vi "PDP.vi"() -> ()   [LabVIEW 2019]
doc: "This VI represents about 90% of the user interface, the remainder consisting of the various pop-up windows.\nA diagram of the NMR system is presented, with buttons to represent each component. Parameters may be changed by pressing one of these buttons, which results in messages being passed to one of several other, high-level VIs whose job it is to take action. After such action is taken, messages may be passed back to this VI, indicating new data to be displayed on the front panel."
uses:
  PDP Global.vi
  TPS Global.vi
  <vilib>/Utility/config.llb/Read Key (Path).vi
  <vilib>/Utility/config.llb/NI_LVConfig.lvlib
panel:
  in  "sel_auto_sw":bool[](array[boolean])=[TRUE, TRUE, TRUE, FALSE, FALSE, FALSE]
  in  "auto_switch_NMR_chan":bool caption="NMR channel \nauto switching"
  in  "RF Off":bool
  in  "RF On":bool
  in  "Mon. Time":i32=30
  out "Polysub Signal":cluster{"x-Axis":dbl[], "Signal":dbl[]}(graph)
  out "CarbGlass":dbl=9.54
  out "Bottom Chip":dbl=9.54
  out "Top Chip":dbl=9.54
  out "NMR Tune Light":bool
  in  "NMR Tune":bool
  out "Clear Message Time":i32
  in  "DC Convert":bool
  out "Bot Plat (K)":dbl=nan format="%.1f"
  out "Top Plat (K)":dbl=nan format="%.1f"
  in  "Submit Comment":bool
  in  "User Comment (press submit when done)":string
  in  "Stop NMR Sweep":bool
  in  "Enable TCL Buttons":bool
  in  "NewEventFile":bool
  in  "NewBaseFile":bool
  out "Separator Flow":dbl=10.0 format="%.1f"
  out "Main Flow":dbl=9.83 format="%.1f"
  in  "Beep on Update":bool
  out "Raw & Base":cluster{"x-Axis":dbl[], "Signal":dbl[]}[](graph)
  in  "5 min":bool
  out "History Plot":cluster{dbl, dbl}[](graph)
  out "Event Number":i32=-15
  in  "Scan Freq":i32=100
  in  "ScanSteps":i32=500
  in  "RF Power":i32=280
  in  "RF Mod":i32=400
  in  "Sweeps":i32=100
  in  "RF Freq":dbl=213.0 format="%.3f"
  in  "Yale Gain":i32(listbox)
  in  "Decrease":bool
  in  "Increase":bool
  in  "Up":bool
  in  "Down":bool
  in  "+1 hour":bool
  in  "30 min":bool
  in  "15 min":bool
  out "Polarization (%)":string="-13.06%"
  out "Monitor Light":bool
  in  "Monitor":bool
  out "Take Data Light":bool
  out "Pause Light":bool=TRUE
  out "QMeter":string="Bot Proton NH3"
  in  "Error":bool
  out "3He Pressure":dbl=9.83 format="%.3f"
  out "4He Pressure":dbl=-0.06 format="%.3f"
  out "Timestamp":string="06May1999  19h28m14s"
  in  "Init QCA":bool
  out "PolyFit Area (arb units)":dbl=-14.751 format="%.8f"
  out "User Message":string="Message: 23Jul2001  15h39m59s\nQCA Module Started"
  in  "Cal. Const.":dbl=0.64413 format="%.6f"
  out "Update At (sec)":dbl=2147483647.0
  out "Next Update":dbl=1151566443.0 format="%.1f"
  in  "Baseline":bool
  out "Subtracted Signal & PolyFit Curve":cluster{"x-Axis":dbl[], "Signal":dbl[]}[](graph)
  out "3He Temp":dbl=1.023 format="%.2f"
  out "4He Temp":dbl=nan format="%.2f"
  in  "Save Channel List":bool
  in  "NMR Channel":i32(listbox)
  in  "Previous Messages":u16(ring)
  in  "Take Data":bool
  in  "One Point":bool
  in  "Pause":bool
  # "PDP:  Polarization Display Panel"
  # "Data for Last Event Displayed:"
  # "RF Output"
  # "X-Axis"
  # "Temp (K)"
  # "Press (Torr)"
  # "4He"
  # "Y-Axis"
  # "3He"
  # "Top"
  # "Bottom"
  # "Chip (W)"
  # "Plat (K)"
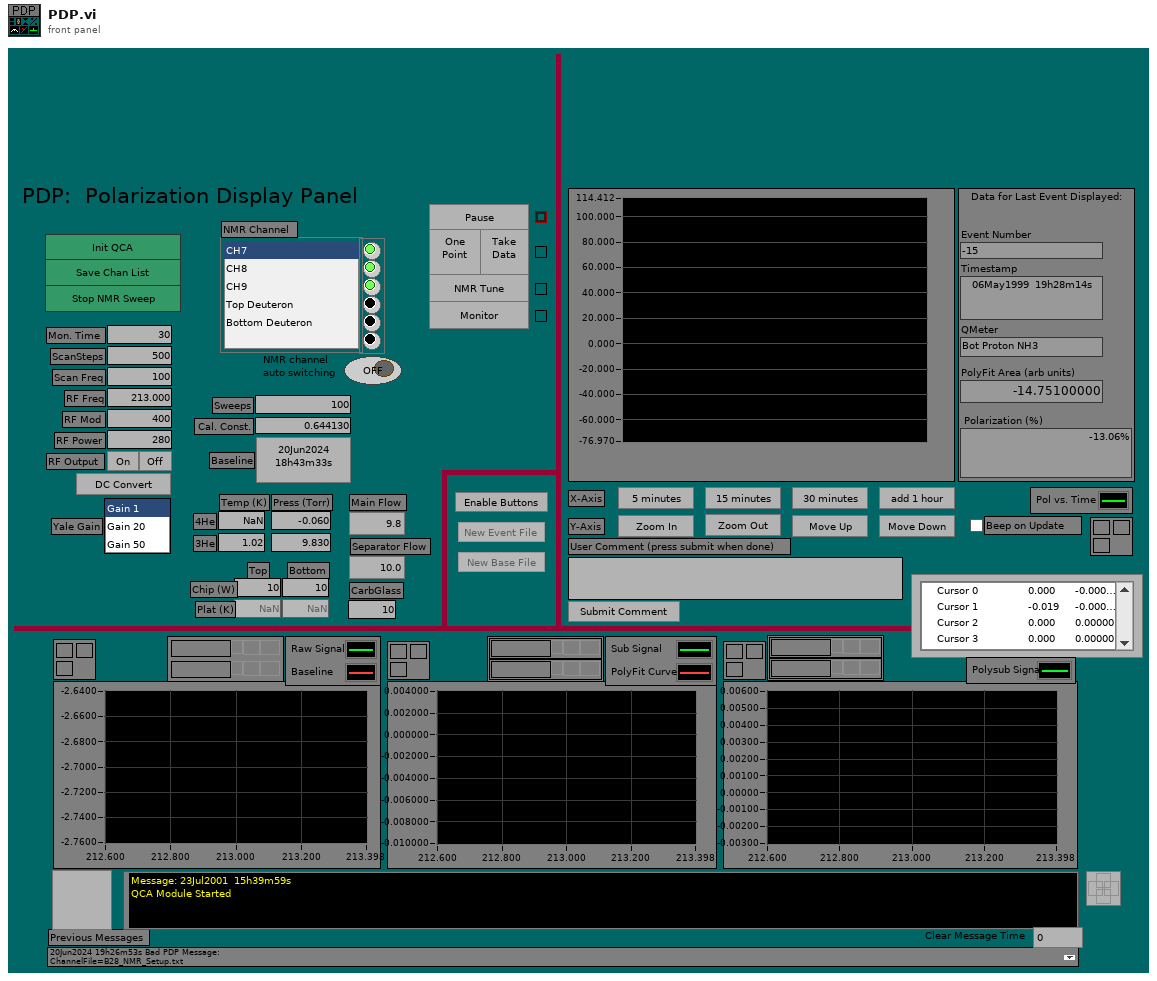
[diagram p1: front panel]
types:
  T1 = enum16{"No Message", "Bad Message", "RFFreq=", "RFMod=", "RFPower=", "QMeterName=", "YaleGain=", "ScanSweeps=", "ScanSteps=", "ScanFreq=", "Material=", "Baseline=", "CalConst=", "MonitorDelay=", "Channel=", "Channels=", "QCAPause", "QCATakeData", "QCANMRTune", "QCAMonitor", "Timer=", "LeadCurrent=", "LeadVoltage=", "MagCurrent=", "MagField=", "MagStatus=", "Setpoint=", "Setrate=", "HeaterDelay=", "Heater=", "HeaterDialog", "MagRemote", "MagLocal", "SendHe4Range", "uWaveFreq=", "uWavePower=", "BellowsPos=", "Event=", "Beep", "Message=", "Warning=", "Error=", "Address=", "Stop"}
  T2 = typedef "NI_LVConfig.lvlib/Config Data RefNum.ctl" = refnum<k1>
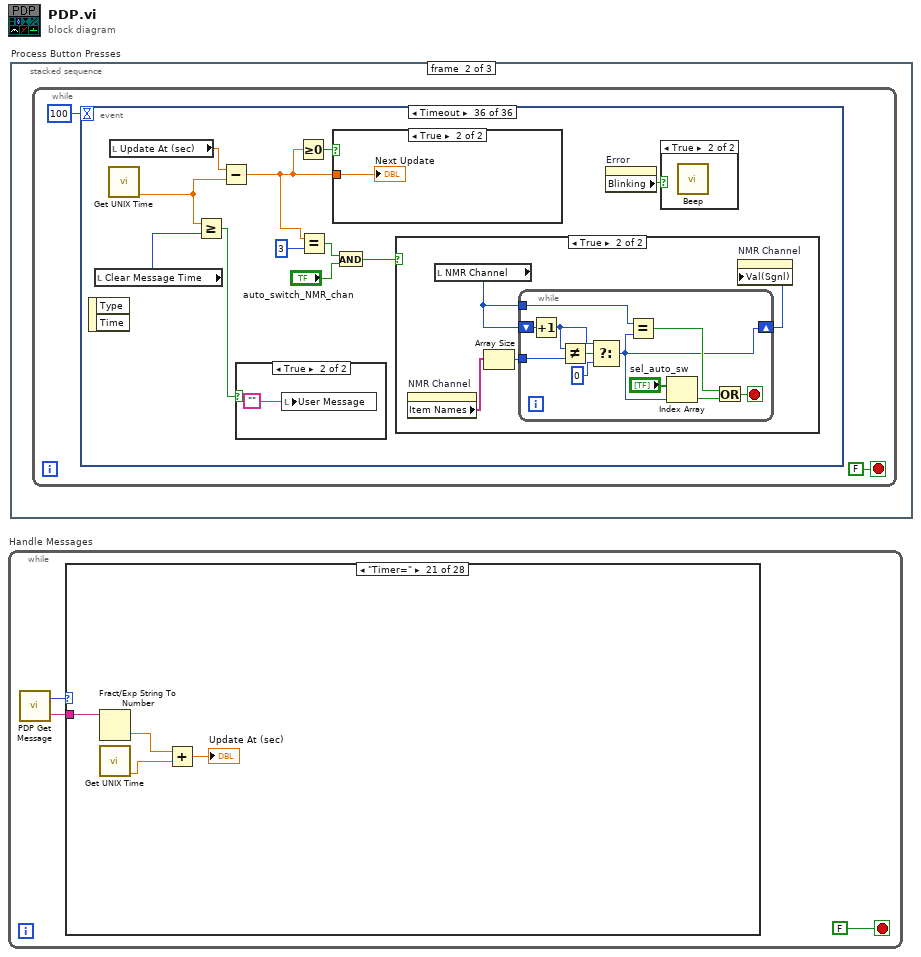
[diagram p0: block diagram]
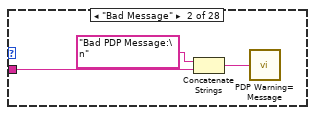
[diagram p3: hidden frame]
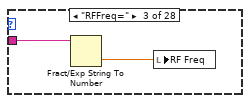
[diagram p4: hidden frame]
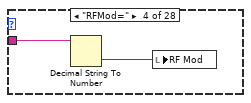
[diagram p5: hidden frame]
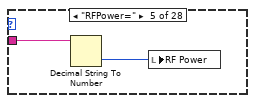
[diagram p6: hidden frame]
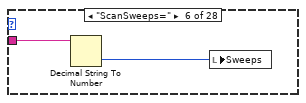
[diagram p7: hidden frame]
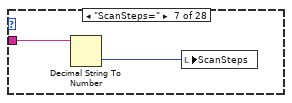
[diagram p8: hidden frame]
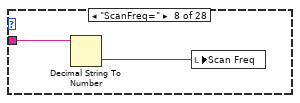
[diagram p9: hidden frame]
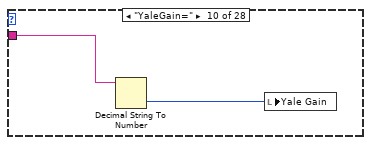
[diagram p11: hidden frame]
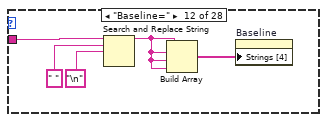
[diagram p13: hidden frame]
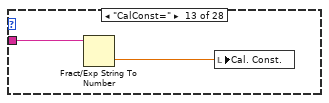
[diagram p14: hidden frame]
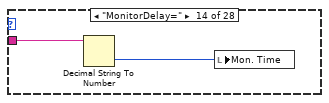
[diagram p15: hidden frame]
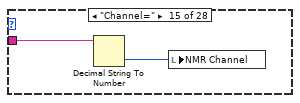
[diagram p16: hidden frame]
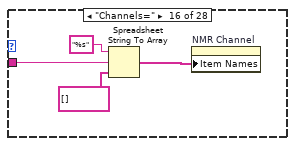
[diagram p17: hidden frame]
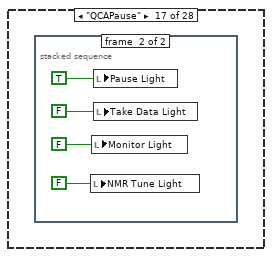
[diagram p18: hidden frame]
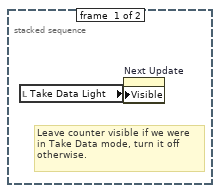
[diagram p19: hidden frame]
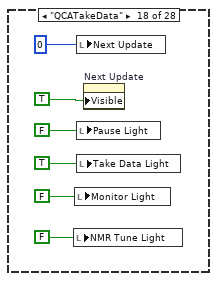
[diagram p20: hidden frame]
diagram:
  n1 = while "Handle Messages" {
    stop <- FALSE stop-if-true
    n2 = call "PDP Get Message.vi"() -> ("PDP Message Type"=w2:T1, "Text"=w3:string)  [unwired: 1 in]
    n3 = case shown="\"Timer=\"" w2 {
      tunnel: w3 -> [_ w4 w8 w10 w12 w14 w16 w18 _ w20 _ w24 w27 w29 w31 w32 _ _ _ _ w61 w62 _ w256 w270 w285 w298 _]
      frame "No Message", Default {
      }
      frame "Bad Message" {
        n4 = Concatenate Strings("Bad PDP Message:\n" ("Message"), w4) -> (w5:string)
        n5 = call "PDP Warning= Message.vi"("Message"=w5) -> ()
      }
      frame "RFFreq=" {
        n6 = Fract/Exp String To Number(string=w8) -> (number=w7:dbl)  [unwired: 3 in, 1 out]
        n7 = local write "RF Freq"(w7) -> ()
      }
      frame "RFMod=" {
        n8 = Decimal String To Number(string=w10) -> (number=w9:i32)  [unwired: 2 in, 1 out]
        n9 = local write "RF Mod"(w9) -> ()
      }
      frame "RFPower=" {
        n10 = Decimal String To Number(string=w12) -> (number=w11:i32)  [unwired: 2 in, 1 out]
        n11 = local write "RF Power"(w11) -> ()
      }
      frame "ScanSweeps=" {
        n12 = Decimal String To Number(string=w14) -> (number=w13:i32)  [unwired: 2 in, 1 out]
        n13 = local write "Sweeps"(w13) -> ()
      }
      frame "ScanSteps=" {
        n14 = Decimal String To Number(string=w16) -> (number=w15:i32)  [unwired: 2 in, 1 out]
        n15 = local write "ScanSteps"(w15) -> ()
      }
      frame "ScanFreq=" {
        n16 = Decimal String To Number(string=w18) -> (number=w17:i32)  [unwired: 2 in, 1 out]
        n17 = local write "Scan Freq"(w17) -> ()
      }
      frame "QMeterName=" {
      }
      frame "YaleGain=" {
        n18 = Decimal String To Number(string=w20) -> (number=w19:i32)  [unwired: 2 in, 1 out]
        n19 = local write "Yale Gain"(w19) -> ()
      }
      frame "Material=" {
      }
      frame "Baseline=" {
        n20 = Search and Replace String(input string=w24, search string=" ", replace string="\n" ("replace string (\"\")")) -> (result string=w21:string)  [unwired: 5 in, 3 out]
        n21 = Build Array(w21, w21, w21, w21) -> (w25:string[])
        n22 = property on="Baseline" class="Bool"("Strings [4]"=w25) -> ()  [unwired: 2 in, 2 out]
      }
      frame "CalConst=" {
        n23 = Fract/Exp String To Number(string=w27) -> (number=w26:dbl)  [unwired: 3 in, 1 out]
        n24 = local write "Cal. Const."(w26) -> ()
      }
      frame "MonitorDelay=" {
        n25 = Decimal String To Number(string=w29) -> (number=w28:i32)  [unwired: 2 in, 1 out]
        n26 = local write "Mon. Time"(w28) -> ()
      }
      frame "Channel=" {
        n27 = Decimal String To Number(string=w31) -> (number=w30:i32)  [unwired: 2 in, 1 out]
        n28 = local write "NMR Channel"(w30) -> ()
      }
      frame "Channels=" {
        n29 = Spreadsheet String To Array(format string="%s", spreadsheet string=w32, array type (2D Dbl)=string[] []) -> (array=w34:string[])  [unwired: 1 in]
        n30 = property on="NMR Channel" class="LstBox (strict)"("Item Names"=w34) -> ()  [unwired: 2 in, 2 out]
      }
      frame "QCAPause" {
        n31 = stacked-sequence {
          frame #0 {
            # "Leave counter visible if we were\nin Take Data mode, turn it off\notherwise."
            n32 = local read "Take Data Light"() -> (w36:bool)
            n33 = property on="Next Update" class="DigNum (strict)"("Visible"=w36) -> ()  [unwired: 2 in, 2 out]
          }
          frame #1 {
            n34 = local write "NMR Tune Light"(FALSE ("NMR Tune Light")) -> ()
            n35 = local write "Monitor Light"(FALSE ("Cont Sweep Light")) -> ()
            n36 = local write "Pause Light"(TRUE ("Pause Light")) -> ()
            n37 = local write "Take Data Light"(FALSE ("Take Data Light")) -> ()
          }
        }
      }
      frame "QCATakeData" {
        n38 = local write "NMR Tune Light"(FALSE ("NMR Tune Light")) -> ()
        n39 = local write "Monitor Light"(FALSE ("Cont Sweep Light")) -> ()
        n40 = local write "Next Update"(0 ("Next Update")) -> ()
        n41 = local write "Pause Light"(FALSE ("Pause Light")) -> ()
        n42 = local write "Take Data Light"(TRUE ("Take Data Light")) -> ()
        n43 = property on="Next Update" class="DigNum (strict)"("Visible"=TRUE) -> ()  [unwired: 2 in, 2 out]
      }
      frame "QCANMRTune" {
        n44 = local write "NMR Tune Light"(TRUE ("NMR Tune Light")) -> ()
        n45 = local write "Monitor Light"(FALSE ("Cont Sweep Light")) -> ()
        n46 = local write "Pause Light"(FALSE ("Pause Light")) -> ()
        n47 = local write "Take Data Light"(FALSE ("Take Data Light")) -> ()
        n48 = property on="Next Update" class="DigNum (strict)"("Visible"=FALSE) -> ()  [unwired: 2 in, 2 out]
      }
      frame "QCAMonitor" {
        n49 = local write "NMR Tune Light"(FALSE ("NMR Tune Light")) -> ()
        n50 = local write "Monitor Light"(TRUE ("Cont Sweep Light")) -> ()
        n51 = local write "Next Update"(0 ("Next Update")) -> ()
        n52 = local write "Pause Light"(FALSE ("Pause Light")) -> ()
        n53 = local write "Take Data Light"(FALSE ("Take Data Light")) -> ()
        n54 = property on="Next Update" class="DigNum (strict)"("Visible"=TRUE) -> ()  [unwired: 2 in, 2 out]
      }
      frame "Timer=" {
        n55 = Fract/Exp String To Number(string=w61) -> (number=w60:dbl)  [unwired: 3 in, 1 out]
        n56 = call "Get UNIX Time.vi"() -> ("UNIX_seconds_dbl"=w58:dbl)  [unwired: 10 in, 1 out]
        n57 = Add(x=w60, y=w58) -> (x+y=→"Update At (sec)":dbl)
      }
      frame "Event=" {
        n58 = Unflatten From String(type=string[][] [], binary string=w62) -> (value=w64:string[][])  [unwired: 3 in, 2 out]
        n59 = stacked-sequence {
          tunnel: w64 -> [w75 w103 w124 w131 w134 w138 w165 w168 w173 w177 w181 w186 w197 w206 w209 w215 w224 w233 w237 w243 _ w251]
          frame #0 {
            # "Set the X axis of the signal plots."
            n60 = call "Text Get Event Fragment.vi"("Event"=w75, "Fragment Type"="RFFreq") -> ("Fragment"=w80:string)  [unwired: 1 out]
            n61 = call "Text Get Event Fragment.vi"("Event"=w75, "Fragment Type"="RFMod") -> ("Fragment"=w81:string)  [unwired: 1 out]
            n62 = call "Text Get Event Fragment.vi"("Event"=w75, "Fragment Type"="ScanSteps") -> ("Fragment"=w77:string)  [unwired: 1 out]
            n63 = global read "PDP Global.vi" "Last Mod"() -> (w71:dbl)
            n64 = global read "PDP Global.vi" "Last Freq"() -> (w74:dbl)
            n65 = global read "PDP Global.vi" "Last Steps"() -> (w72:i32)
            n66 = Fract/Exp String To Number(string=w80) -> (number=w73:dbl)  [unwired: 3 in, 1 out]
            n67 = Decimal String To Number(string=w81) -> (number=w79:i32)  [unwired: 2 in, 1 out]
            n68 = Decimal String To Number(string=w77) -> (number=w69:i32)  [unwired: 2 in, 1 out]
            n69 = Divide(x=w79, y=1000) -> (x/y=w70:dbl)
            n70 = Not Equal?(x=w74, y=w73) -> (x != y?=w66:bool)
            n71 = Not Equal?(x=w71, y=w70) -> (x != y?=w67:bool)
            n72 = Not Equal?(x=w72, y=w69) -> (x != y?=w68:bool)
            n73 = Compound Arithmetic op=OR(w66, w67, w68) -> (w65:bool)
            n74 = case shown="True" w65 {
              tunnel: w69 -> [_ w86]
              tunnel: w70 -> [_ w85]
              tunnel: w73 -> [_ w84]
              frame False {
              }
              frame True {
                n75 = global write "PDP Global.vi" "Last Mod"(w85) -> ()
                n76 = global write "PDP Global.vi" "Last Freq"(w84) -> ()
                n77 = global write "PDP Global.vi" "Last Steps"(w86) -> ()
                n78 = for {
                  N: w86 -> [_]
                  tunnel: [w94] -> w89 mode=indexing
                  i -> [w94]
                }
                n79 = Multiply(x=w89, y=2) -> (x*y=w90:i32[])
                n80 = Divide(x=w90, y=w86) -> (x/y=w93:dbl[])
                n81 = Decrement(x=w93) -> (x-1=w87:dbl[])
                n82 = Multiply(x=w85, y=w87) -> (x*y=w92:dbl[])
                n83 = Add(x=w84, y=w92) -> (x+y=w91:dbl[])
                n84 = global write "PDP Global.vi" "x-Axis"(w91) -> ()
              }
            }
          }
          frame #1 {
            # "Display the Raw Signal and the Baseline Signal."
            n85 = call "Text Get Event Fragment.vi"("Event"=w103, "Fragment Type"="RawSignal") -> ("Fragment"=w102:string)  [unwired: 1 out]
            n86 = call "Text Get Event Fragment.vi"("Event"=w103, "Fragment Type"="BaseSignal") -> ("Fragment"=w101:string)  [unwired: 1 out]
            n87 = global read "PDP Global.vi" "x-Axis"() -> (w99:dbl[])
            n88 = call "String 2 Signal.vi"("String"=w102) -> ("Signal"=w96:dbl[])
            n89 = call "String 2 Signal.vi"("String"=w101) -> ("Signal"=w98:dbl[])
            n90 = Array Size(array=w98) -> (size(s)=w100:i32)
            n91 = Greater Than 0?(x=w100) -> (x > 0?=w95:bool)
            n92 = case shown="True" w95 {
              tunnel: w99 -> [w109 w110]
              tunnel: w98 -> [_ w115]
              tunnel: [w106 w112] -> w97
              tunnel: w96 -> [w108 w111]
              frame False {
                n93 = Bundle("x-Axis"=w109, "Signal"=w108) -> (w107:cluster{"x-Axis":dbl[], "Signal":dbl[]})  [unwired: 1 in]
                n94 = Build Array(w107) -> (w106:cluster{"x-Axis":dbl[], "Signal":dbl[]}[])
              }
              frame True {
                n95 = Bundle("x-Axis"=w110, "Signal"=w111) -> (w114:cluster{"x-Axis":dbl[], "Signal":dbl[]})  [unwired: 1 in]
                n96 = Bundle("x-Axis"=w110, "Signal"=w115) -> (w113:cluster{"x-Axis":dbl[], "Signal":dbl[]})  [unwired: 1 in]
                n97 = Build Array(w114, w113) -> (w112:cluster{"x-Axis":dbl[], "Signal":dbl[]}[])
              }
            }
            "Raw & Base" <- w97
          }
          frame #2 {
            # "Display the Subtracted Signal and the Polyfit Curve."
            n98 = call "Text Get Event Fragment.vi"("Event"=w124, "Fragment Type"="SubSignal") -> ("Fragment"=w122:string)  [unwired: 1 out]
            n99 = call "Text Get Event Fragment.vi"("Event"=w124, "Fragment Type"="PolyCurve") -> ("Fragment"=w123:string)  [unwired: 1 out]
            n100 = global read "PDP Global.vi" "x-Axis"() -> (w119:dbl[])
            n101 = call "String 2 Signal.vi"("String"=w122) -> ("Signal"=w116:dbl[])
            n102 = call "String 2 Signal.vi"("String"=w123) -> ("Signal"=w120:dbl[])
            n103 = Bundle("x-Axis"=w119, "Signal"=w116) -> (w117:cluster{"x-Axis":dbl[], "Signal":dbl[]})  [unwired: 1 in]
            n104 = Bundle("x-Axis"=w119, "Signal"=w120) -> (w118:cluster{"x-Axis":dbl[], "Signal":dbl[]})  [unwired: 1 in]
            n105 = Build Array(w117, w118) -> (→"Subtracted Signal & PolyFit Curve":cluster{"x-Axis":dbl[], "Signal":dbl[]}[])
          }
          frame #3 {
            # "Display the Polysubtracted Signal."
            n106 = call "Text Get Event Fragment.vi"("Event"=w131, "Fragment Type"="PolySignal") -> ("Fragment"=w128:string)  [unwired: 1 out]
            n107 = global read "PDP Global.vi" "x-Axis"() -> (w130:dbl[])
            n108 = call "String 2 Signal.vi"("String"=w128) -> ("Signal"=w127:dbl[])
            n109 = Bundle("x-Axis"=w130, "Signal"=w127) -> (→"Polysub Signal":cluster{"x-Axis":dbl[], "Signal":dbl[]})  [unwired: 1 in]
          }
          frame #4 {
            # "Display the Polysubtracted Signal."
            n110 = call "Text Get Event Fragment.vi"("Event"=w134, "Fragment Type"="Area") -> ("Fragment"=w135:string)  [unwired: 1 out]
            n111 = Fract/Exp String To Number(string=w135) -> (number=→"PolyFit Area (arb units)":dbl)  [unwired: 3 in, 1 out]
          }
          frame #5 {
            # "Display the Polysubtracted Signal."
            n112 = call "Text Get Event Fragment.vi"("Event"=w138, "Fragment Type"="Polarization") -> ("Fragment"=w144:string, "Found"=w137:bool)
            n113 = call "Text Get Event Fragment.vi"("Event"=w138, "Fragment Type"="EventNum") -> ("Fragment"=w140:string)  [unwired: 1 out]
            n114 = Decimal String To Number(string=w140) -> (number=w139:i32)  [unwired: 2 in, 1 out]
            n115 = Fract/Exp String To Number(string=w144) -> (number=w142:dbl)  [unwired: 3 in, 1 out]
            n116 = case shown="True" w137 {
              tunnel: w142 -> [_ w146]
              tunnel: w139 -> [_ w150]
              frame False {
                n117 = local write "Polarization (%)"("") -> ()
              }
              frame True {
                n118 = call "UNIX to LabVIEW.vi"("UNIX Time"=w150) -> ("LabVIEW Time"=w151:dbl)
                n119 = Absolute Value(x=w146) -> (abs(x)=w149:dbl)
                n120 = property on="History Plot" class="XYGraph (strict)"() -> ("X Scale.Range:Maximum"=w154:dbl, "X Scale.Range:Minimum"=w157:dbl)  [unwired: 2 in, 2 out]
                n121 = Less?(x=w149, y=101.0) -> (x < y?=w147:bool)
                n122 = Format Into String(format string="%+6.1f%", w146) -> (resulting string=→"Polarization (%)":string)  [unwired: 2 in, 1 out]
                n123 = case shown="True" w147 {
                  tunnel: w151 -> [_ w160]
                  tunnel: w146 -> [_ w159]
                  frame False {
                    # "Glitch Signal - don't plot in strip chart"
                  }
                  frame True {
                    n124 = local read "History Plot"() -> (w163:cluster{dbl, dbl}[])
                    n125 = Bundle("LabVIEW Time"=w160, w159) -> (w161:cluster{"LabVIEW Time":dbl, dbl})  [unwired: 1 in]
                    n126 = Build Array (concatenate)(w161, w163) -> (→"History Plot":cluster{"LabVIEW Time":dbl, dbl}[])
                  }
                }
                n127 = Subtract(x=w151, y=w154) -> (x-y=w158:dbl)
                n128 = Compound Arithmetic op=ADD(w158, w154) -> (w156:dbl)
                n129 = Compound Arithmetic op=ADD(w158, w157) -> (w155:dbl)
                n130 = property on="History Plot" class="XYGraph (strict)"("X Scale.Range:Maximum"=w156, "X Scale.Range:Minimum"=w155) -> ()  [unwired: 2 in, 2 out]
              }
            }
          }
          frame #6 {
            # "Display the Polysubtracted Signal."
            n131 = call "Text Get Event Fragment.vi"("Event"=w165, "Fragment Type"="QMeterName") -> ("Fragment"=→"QMeter":string)  [unwired: 1 out]
          }
          frame #7 {
            n132 = call "Text Get Event Fragment.vi"("Event"=w168, "Fragment Type"="EventNum") -> ("Fragment"=w169:string)  [unwired: 1 out]
            n133 = Decimal String To Number(string=w169) -> (number=w167:i32)  [unwired: 2 in, 1 out]
            "Event Number" <- w167
            n134 = call "UNIX to Timestamp.vi"("Seconds"=w167) -> ("Timestamp String"=→"Timestamp":string)
          }
          frame #8 {
            # "Display the Polysubtracted Signal."
            n135 = call "Text Get Event Fragment.vi"("Event"=w173, "Fragment Type"="He3Press") -> ("Fragment"=w174:string)  [unwired: 1 out]
            n136 = Fract/Exp String To Number(string=w174) -> (number=→"3He Pressure":dbl)  [unwired: 3 in, 1 out]
          }
          frame #9 {
            # "Display the Polysubtracted Signal."
            n137 = call "Text Get Event Fragment.vi"("Event"=w177, "Fragment Type"="He3Temp") -> ("Fragment"=w178:string)  [unwired: 1 out]
            n138 = Fract/Exp String To Number(string=w178) -> (number=→"3He Temp":dbl)  [unwired: 3 in, 1 out]
          }
          frame #10 {
            # "Display the Polysubtracted Signal."
            n139 = call "Text Get Event Fragment.vi"("Event"=w181, "Fragment Type"="He4Press") -> ("Fragment"=w182:string)  [unwired: 1 out]
            n140 = Fract/Exp String To Number(string=w182) -> (number=→"4He Pressure":dbl)  [unwired: 3 in, 1 out]
          }
          frame #11 {
            # "Display the Polysubtracted Signal."
            n141 = call "Text Get Event Fragment.vi"("Event"=w186, "Fragment Type"="He4Temp") -> ("Fragment"=w187:string, "Found"=w184:bool)
            n142 = Fract/Exp String To Number(string=w187) -> (number=w185:dbl)  [unwired: 3 in, 1 out]
            n143 = case shown="True" w184 {
              tunnel: w185 -> [_ w189]
              frame False {
              }
              frame True {
                "4He Temp" <- w189
              }
            }
          }
          frame #12 {
            # "Display the Polysubtracted Signal."
            n144 = call "Text Get Event Fragment.vi"("Event"=w197, "Fragment Type"="TopPlat") -> ("Fragment"=w192:string)  [unwired: 1 out]
            n145 = Fract/Exp String To Number(string=w192) -> (number=w191:dbl)  [unwired: 3 in, 1 out]
            "Top Plat (K)" <- w191
            n146 = Less?(x=w191, y=49.0) -> (x < y?=w196:bool)
            n147 = Select(t=2, s=w196, f=0) -> (s? t:f=w193:i32)
            n148 = property on="Top Plat (K)" class="DigNum (strict)"("Disabled"=w193) -> ()  [unwired: 2 in, 2 out]
          }
          frame #13 {
            # "Display the Polysubtracted Signal."
            n149 = call "Text Get Event Fragment.vi"("Event"=w206, "Fragment Type"="BotPlat") -> ("Fragment"=w202:string)  [unwired: 1 out]
            n150 = Fract/Exp String To Number(string=w202) -> (number=w199:dbl)  [unwired: 3 in, 1 out]
            "Bot Plat (K)" <- w199
            n151 = Less?(x=w199, y=49.0) -> (x < y?=w205:bool)
            n152 = Select(t=2, s=w205, f=0) -> (s? t:f=w200:i32)
            n153 = property on="Bot Plat (K)" class="DigNum (strict)"("Disabled"=w200) -> ()  [unwired: 2 in, 2 out]
          }
          frame #14 {
            n154 = call "Text Get Event Fragment.vi"("Event"=w209, "Fragment Type"="MainFlow") -> ("Fragment"=w210:string)  [unwired: 1 out]
            n155 = Fract/Exp String To Number(string=w210) -> (number=→"Main Flow":dbl)  [unwired: 3 in, 1 out]
          }
          frame #15 {
            n156 = call "Text Get Event Fragment.vi"("Event"=w215, "Fragment Type"="SepFlow") -> ("Fragment"=w216:string)  [unwired: 1 out]
            n157 = Fract/Exp String To Number(string=w216) -> (number=w213:dbl)  [unwired: 3 in, 1 out]
            "Separator Flow" <- w213
            n158 = Less?(x=w213, y=7.0) -> (x < y?=w214:bool)
            n159 = property on="Separator Flow" class="DigNum (strict)"("Blinking"=w214) -> ()  [unwired: 2 in, 2 out]
          }
          frame #16 {
            w223 = 1300  # Liquid Threshold
            n160 = call "Text Get Event Fragment.vi"("Event"=w224, "Fragment Type"="TopChip") -> ("Fragment"=w225:string)  [unwired: 1 out]
            n161 = Fract/Exp String To Number(string=w225) -> (number=w222:dbl)  [unwired: 3 in, 1 out]
            "Top Chip" <- w222
            n162 = Greater?(x=w222, y=w223) -> (0:w219:bool)
            n163 = Select(t=u32 4372735, s=w219, f=u32 11776947) -> (s? t:f=w218:u32)
            n164 = property on="Top Chip" class="DigNum (strict)"("Numeric Text.Text Colors:BG Color"=w218) -> ()  [unwired: 2 in, 2 out]
          }
          frame #17 {
            w232 = 1300  # Liquid Threshold
            n165 = call "Text Get Event Fragment.vi"("Event"=w233, "Fragment Type"="BottomChip") -> ("Fragment"=w234:string)  [unwired: 1 out]
            n166 = Fract/Exp String To Number(string=w234) -> (number=w231:dbl)  [unwired: 3 in, 1 out]
            "Bottom Chip" <- w231
            n167 = Greater?(x=w231, y=w232) -> (0:w228:bool)
            n168 = Select(t=u32 4372735, s=w228, f=u32 11776947) -> (s? t:f=w227:u32)
            n169 = property on="Bottom Chip" class="DigNum (strict)"("Numeric Text.Text Colors:BG Color"=w227) -> ()  [unwired: 2 in, 2 out]
          }
          frame #18 {
            n170 = call "Text Get Event Fragment.vi"("Event"=w237, "Fragment Type"="CarbonGlass") -> ("Fragment"=w238:string)  [unwired: 1 out]
            n171 = Fract/Exp String To Number(string=w238) -> (number=→"CarbGlass":dbl)  [unwired: 3 in, 1 out]
          }
          frame #19 {
            n172 = call "Text Get Event Fragment.vi"("Event"=w243, "Fragment Type"="VacPress") -> ("Fragment"=w244:string)  [unwired: 1 out]
            n173 = Fract/Exp String To Number(string=w244) -> (number=w242:dbl)  [unwired: 3 in, 1 out]
            n174 = Power Of 10(x=w242) -> (10^x=w241:dbl)
            n175 = Greater?(x=w241, y=5e-05) -> ()  [unwired: 1 out]
          }
          frame #20 {
            n176 = case shown="True" "Beep on Update" {
              frame False {
              }
              frame True {
                n177 = call <vilib>:"Beep.vi"() -> ()  [unwired: 12 in]
              }
            }
          }
          frame #21 {
            # "Tell the event builder that we're done."
            n178 = call "Text Get Event Fragment.vi"("Event"=w251, "Fragment Type"="EventNum") -> ("Fragment"=w249:string)  [unwired: 1 out]
            n179 = Decimal String To Number(string=w249) -> (number=w248:i32)  [unwired: 2 in, 1 out]
            n180 = call "TEB Processed= Message.vi"("Module Name"="PDP", "Event Number"=w248) -> ()
          }
        }
      }
      frame "Beep" {
        n181 = call <vilib>:"Beep.vi"() -> ()  [unwired: 12 in]
      }
      frame "Message=" {
        n182 = call "Get UNIX Time.vi"() -> ("UNIX seconds"=w253:i32)  [unwired: 10 in, 1 out]
        n183 = call "UNIX to Timestamp.vi"("Seconds"=w253) -> ("Timestamp String"=w265:string)
        n184 = Add(x=60, y=w253) -> (x+y=→"Clear Message Time":i32)
        n185 = property on="Previous Messages" class="Ring (strict)"() -> ("Strings []"=w259:string[])  [unwired: 2 in, 2 out]
        n186 = Format Into String(format string="Message: %s\n%s", w265, w256) -> (resulting string=w255:string)  [unwired: 2 in, 1 out]
        n187 = Format Into String(format string="%s %s", w265, w256) -> (resulting string=w264:string)  [unwired: 2 in, 1 out]
        n188 = Array Subset(array=w259, length=99) -> (w261:string[])  [unwired: 1 in]
        n189 = Build Array (concatenate)(w264, w261) -> (w262:string[])
        n190 = local write "User Message"(w255) -> ()
        n191 = call "PDP Log Message.vi"("Message"=w255) -> ()
        n192 = property on="Previous Messages" class="Ring (strict)"("Strings []"=w262) -> ()  [unwired: 2 in, 2 out]
        n193 = property on="User Message" class="Str"("Text.Text Colors:Text Color"=u32 65280) -> ()  [unwired: 2 in, 2 out]
      }
      frame "Warning=" {
        n194 = call "Get UNIX Time.vi"() -> ("UNIX seconds"=w267:i32)  [unwired: 10 in, 1 out]
        n195 = Add(x=180, y=w267) -> (x+y=w268:i32)
        n196 = call "UNIX to Timestamp.vi"("Seconds"=w267) -> ("Timestamp String"=w279:string)
        n197 = local write "Clear Message Time"(w268) -> ()
        n198 = property on="Previous Messages" class="Ring (strict)"() -> ("Strings []"=w273:string[])  [unwired: 2 in, 2 out]
        n199 = Format Into String(format string="Warning: %s\n%s", w279, w270) -> (resulting string=w269:string)  [unwired: 2 in, 1 out]
        n200 = Format Into String(format string="%s %s", w279, w270) -> (resulting string=w278:string)  [unwired: 2 in, 1 out]
        n201 = Array Subset(array=w273, length=99) -> (w275:string[])  [unwired: 1 in]
        n202 = Build Array (concatenate)(w278, w275) -> (w276:string[])
        n203 = local write "User Message"(w269) -> ()
        n204 = call "PDP Log Message.vi"("Message"=w269) -> ()
        n205 = property on="Previous Messages" class="Ring (strict)"("Strings []"=w276) -> ()  [unwired: 2 in, 2 out]
        n206 = call <vilib>:"Beep.vi"() -> ()  [unwired: 12 in]
        n207 = property on="User Message" class="Str"("Text.Text Colors:Text Color"=u32 16776960) -> ()  [unwired: 2 in, 2 out]
      }
      frame "Error=" {
        n208 = call "Get UNIX Time.vi"() -> ("UNIX seconds"=w281:i32)  [unwired: 10 in, 1 out]
        n209 = Add(x=300, y=w281) -> (x+y=w282:i32)
        n210 = call "UNIX to Timestamp.vi"("Seconds"=w281) -> ("Timestamp String"=w294:string)
        n211 = property on="Previous Messages" class="Ring (strict)"() -> ("Strings []"=w288:string[])  [unwired: 2 in, 2 out]
        n212 = local write "Clear Message Time"(w282) -> ()
        n213 = Format Into String(format string="Error: %s\n%s", w294, w285) -> (resulting string=w283:string)  [unwired: 2 in, 1 out]
        n214 = Format Into String(format string="%s %s", w294, w285) -> (resulting string=w293:string)  [unwired: 2 in, 1 out]
        n215 = Array Subset(array=w288, length=99) -> (w290:string[])  [unwired: 1 in]
        n216 = Build Array (concatenate)(w293, w290) -> (w291:string[])
        n217 = local write "User Message"(w283) -> ()
        n218 = call "PDP Log Message.vi"("Message"=w283) -> ()
        n219 = property on="Previous Messages" class="Ring (strict)"("Strings []"=w291) -> ()  [unwired: 2 in, 2 out]
        n220 = property on="Error" class="Bool (strict)"("Blinking"=TRUE) -> ()  [unwired: 2 in, 2 out]
        n221 = property on="User Message" class="Str"("Text.Text Colors:Text Color"=u32 16711680) -> ()  [unwired: 2 in, 2 out]
      }
      frame "Address=" {
        n222 = Scan From String(format string="%3s,%[.0-9]:%d" ("Format String"), input string=w298) -> (output 1=w296:string, output 2=w297:string, output 3=w295:i32)  [unwired: 5 in, 3 out]
        n223 = call "Message Set Module Address.vi"("Port"=w295, "Address"=w297, "Module"=w296) -> ()
      }
      frame "Stop" {
        n224 = Stop() -> ()  [unwired: 1 in]
      }
    }
  }
  n225 = stacked-sequence "Process Button Presses" {
    frame #0 {
      w300 = TRUE ("X Editable")
      # "Check that the path global has been set."
      # "Perform any necessary startup functions."
      n226 = global read "TPS Global.vi" "TPS Base Path"() -> (w303:path)
      n227 = local write "User Message"("") -> ()
      n228 = property on="Subtracted Signal & PolyFit Curve" class="XYGraph (strict)"("X Scale.Editable"=w300) -> ()  [unwired: 2 in, 2 out]
      n229 = property on="Polysub Signal" class="XYGraph (strict)"("X Scale.Editable"=w300) -> ()  [unwired: 2 in, 2 out]
      n230 = Not A Number/Path/Refnum?(number/path/refnum=w303) -> (NaN/Path/Refnum?=w304:bool)
      n231 = case shown="False" w304 {
        tunnel: w303 -> [w309 _]
        frame False {
          n232 = global read "TPS Global.vi" "TPS Setup File"() -> (w317:string)
          n233 = Build Path(base path=w309, name or relative path=w317) -> (appended path=w316:path)
          n234 = call <vilib>:"Open Config Data (compatibility).vi"("create file if necessary (T)"=FALSE ("create file if necessary? (T)"), "configuration file path"=w316) -> ("error out"=w318:errorcluster, "refnum"=w314:T2)  [unwired: 7 in, 1 out]
          n235 = call-poly <vilib>:"Read Key.vi"("section"="PDP", "error in (no error)"=w318, "default value"=path "", "key"="Message Log", "refnum"=w314) -> ("error out"=w319:errorcluster, "value"=w308:path, "refnum out"=w310:T2)  [unwired: 3 in, 1 out]
          n236 = call <vilib>:"Close Config Data.vi"("error in (no error)"=w319, "write file if changed (T)"=FALSE, "refnum"=w310) -> ("error out"=w320:errorcluster)  [unwired: 7 in, 1 out]
          n237 = Build Path(base path=w309, name or relative path=w308) -> (appended path=w307:path)
          n238 = global write "PDP Global.vi" "Message Log"(w307) -> ()
          n239 = call <vilib>:"Simple Error Handler.vi"("error in (no error)"=w320) -> ()  [unwired: 4 in, 5 out]
        }
        frame True {
          n240 = One Button Dialog(message="The Base Path global has not been set.  Please set it and run again.") -> (true=w322:bool)  [unwired: 1 in]
          n241 = Stop(stop? (T)=w322) -> ()
        }
      }
      n242 = call "Message Send.vi"("Message"="Read", "Destination"="SMC") -> ()
    }
    frame #1 {
      n243 = while {
        stop <- FALSE stop-if-true
        n244 = event shown="[35] Timeout" {
          selector: _ -> [_ _ _ _ _ _ _ _ _ _ _ _ _ _ _ _ _ _ _ _ _ _ _ _ _ _ _ _ _ _ _ _ _ _ _ _]
          dyn-events: _ -> [_ _ _ _ _ _ _ _ _ _ _ _ _ _ _ _ _ _ _ _ _ _ _ _ _ _ _ _ _ _ _ _ _ _ _ _]
          timeout: 100 -> [_ _ _ _ _ _ _ _ _ _ _ _ _ _ _ _ _ _ _ _ _ _ _ _ _ _ _ _ _ _ _ _ _ _ _ _]
          event "Init QCA": Value Change {
            n245 = event-data() -> ()  [unwired: 1 in, 4 out]
            n246 = call "Message Send.vi"("Message"="Init", "Destination"="QCA") -> ()
          }
          event "Save Channel List": Value Change {
            n247 = event-data() -> ()  [unwired: 1 in, 4 out]
            n248 = call "Message Send.vi"("Message"="SaveChans", "Destination"="QCA") -> ()
          }
          event "Stop NMR Sweep": Value Change {
            n249 = event-data() -> ()  [unwired: 1 in, 5 out]
            n250 = call "Stop NMR Sweep.vi"() -> ()  [unwired: 1 in]
          }
          event "DC Convert": Value Change {
            n251 = event-data() -> ()  [unwired: 1 in, 5 out]
            n252 = call "Yale DC Convert.vi"() -> ()  [unwired: 1 in]
          }
          event "Baseline": Value Change {
            n253 = event-data() -> ()  [unwired: 1 in, 4 out]
            n254 = call "Message Send.vi"("Message"="Baseline", "Destination"="QCA") -> ()
          }
          event "Pause": Value Change {
            n255 = event-data() -> ()  [unwired: 1 in, 4 out]
            n256 = call "Message Send.vi"("Message"="Pause", "Destination"="QCA") -> ()
          }
          event "Take Data": Value Change {
            n257 = event-data() -> ()  [unwired: 1 in, 4 out]
            n258 = call "Message Send.vi"("Message"="TakeData", "Destination"="QCA") -> ()
          }
          event "One Point": Value Change {
            n259 = event-data() -> ()  [unwired: 1 in, 4 out]
            n260 = call "Message Send.vi"("Message"="OnePoint", "Destination"="QCA") -> ()
          }
          event "NMR Tune": Value Change {
            n261 = event-data() -> ()  [unwired: 1 in, 4 out]
            n262 = call "Message Send.vi"("Message"="NMRTune", "Destination"="QCA") -> ()
          }
          event "Monitor": Value Change {
            n263 = event-data() -> ()  [unwired: 1 in, 4 out]
            n264 = call "Message Send.vi"("Message"="Monitor", "Destination"="QCA") -> ()
          }
          event "ScanSteps": Value Change {
            n265 = event-data() -> ("NewVal"=w341:i32)  [unwired: 1 in, 4 out]
            n266 = call "Message Send Integer.vi"("Value"=w341, "Parameter"="ScanSteps" ("Message"), "Destination"="QCA") -> ()
          }
          event "Scan Freq": Value Change {
            n267 = event-data() -> ("NewVal"=w344:i32)  [unwired: 1 in, 4 out]
            n268 = call "Message Send Integer.vi"("Value"=w344, "Parameter"="ScanFreq" ("Message"), "Destination"="QCA") -> ()
          }
          event "RF On": Value Change {
            n269 = event-data() -> ()  [unwired: 1 in, 5 out]
            n270 = call "Message Send.vi"("Message"="RF On", "Destination"="QCA") -> ()
          }
          event "RF Off": Value Change {
            n271 = event-data() -> ()  [unwired: 1 in, 5 out]
            n272 = call "Message Send.vi"("Message"="RF Off", "Destination"="QCA") -> ()
          }
          event "RF Freq": Value Change {
            n273 = event-data() -> ("NewVal"=w351:dbl)  [unwired: 1 in, 4 out]
            n274 = call "Message Send Float.vi"("Value"=w351, "Parameter"="RFFreq" ("Message"), "Destination"="QCA") -> ()
          }
          event "RF Mod": Value Change {
            n275 = event-data() -> ("NewVal"=w354:i32)  [unwired: 1 in, 4 out]
            n276 = call "Message Send Integer.vi"("Value"=w354, "Parameter"="RFMod" ("Message"), "Destination"="QCA") -> ()
          }
          event "RF Power": Value Change {
            n277 = event-data() -> ("NewVal"=w357:i32)  [unwired: 1 in, 4 out]
            n278 = call "Message Send Integer.vi"("Value"=w357, "Parameter"="RFPower" ("Message"), "Destination"="QCA") -> ()
          }
          event "NMR Channel": Value Change {
            n279 = event-data() -> ("NewVal"=w360:i32)  [unwired: 1 in, 4 out]
            n280 = call "Message Send Integer.vi"("Value"=w360, "Parameter"="Channel" ("Message"), "Destination"="QCA") -> ()
          }
          event "Sweeps": Value Change {
            n281 = event-data() -> ("NewVal"=w363:i32)  [unwired: 1 in, 4 out]
            n282 = call "Message Send Integer.vi"("Value"=w363, "Parameter"="ScanSweeps" ("Message"), "Destination"="QCA") -> ()
          }
          event "Cal. Const.": Value Change {
            n283 = event-data() -> ("NewVal"=w366:dbl)  [unwired: 1 in, 4 out]
            n284 = call "Message Send Float.vi"("Value"=w366, "Parameter"="CalConst" ("Message"), "Destination"="QCA") -> ()
          }
          event "Yale Gain": Value Change {
            n285 = event-data() -> ("NewVal"=w369:i32)  [unwired: 1 in, 4 out]
            n286 = call "Message Send Integer.vi"("Value"=w369, "Parameter"="YaleGain" ("Message"), "Destination"="QCA") -> ()
          }
          event "Mon. Time": Value Change {
            n287 = event-data() -> ("NewVal"=w372:i32)  [unwired: 1 in, 4 out]
            n288 = call "Message Send Integer.vi"("Value"=w372, "Parameter"="MonitorDelay" ("Message"), "Destination"="QCA") -> ()
          }
          event "Enable TCL Buttons": Value Change {
            w376 = string[] ["Disable Buttons", "Disable Buttons", "Disable Buttons", "Disable Buttons"] ("Array Constant")
            n289 = event-data() -> ()  [unwired: 1 in, 5 out]
            n290 = property on="Enable TCL Buttons" class="Bool"() -> ("Strings [4]"=w379:string[])  [unwired: 2 in, 2 out]
            n291 = Equal?(x=w379, y=w376) -> (x = y?=w378:bool)
            n292 = Select(t=string[] ["Enable Buttons", "Enable Buttons", "Enable Buttons", "Enable Buttons"] ("Array Constant"), s=w378, f=w376) -> (s? t:f=w382:string[])
            n293 = Select(t=2, s=w378, f=0) -> (s? t:f=w375:i32)
            n294 = property on="Enable TCL Buttons" class="Bool"("Strings [4]"=w382) -> ()  [unwired: 2 in, 2 out]
            n295 = property on="NewEventFile" class="Bool"("Disabled"=w375) -> ()  [unwired: 2 in, 2 out]
            n296 = property on="NewBaseFile" class="Bool"("Disabled"=w375) -> ()  [unwired: 2 in, 2 out]
          }
          event "NewEventFile": Value Change {
            n297 = event-data() -> ()  [unwired: 1 in, 5 out]
            n298 = property on="NewBaseFile" class="Bool"() -> ("Disabled"=w384:u8)  [unwired: 2 in, 2 out]
            n299 = Equal To 0?(x=w384) -> (x = 0?=w383:bool)
            n300 = case shown="True" w383 {
              frame False {
              }
              frame True {
                n301 = call "Message Send.vi"("Message"="NewEventFile", "Destination"="TCL") -> ()
              }
            }
          }
          event "NewBaseFile": Value Change {
            n302 = event-data() -> ()  [unwired: 1 in, 5 out]
            n303 = property on="NewBaseFile" class="Bool"() -> ("Disabled"=w388:u8)  [unwired: 2 in, 2 out]
            n304 = Equal To 0?(x=w388) -> (x = 0?=w387:bool)
            n305 = case shown="True" w387 {
              frame False {
              }
              frame True {
                n306 = call "Message Send.vi"("Message"="NewBaseFile", "Destination"="TCL") -> ()
              }
            }
          }
          event "Error": Value Change {
            w392 = FALSE ("Blinking")
            n307 = event-data() -> ()  [unwired: 1 in, 5 out]
            n308 = local write "Error"(w392) -> ()
            n309 = property on="Error" class="Bool (strict)"("Blinking"=w392) -> ()  [unwired: 2 in, 2 out]
            "User Message" <- ""
          }
          event "5 min": Value Change {
            n310 = event-data() -> ()  [unwired: 1 in, 5 out]
            n311 = property on="History Plot" class="XYGraph (strict)"() -> ("X Scale.Range:Maximum"=w395:dbl)  [unwired: 2 in, 2 out]
            n312 = Subtract(x=w395, y=300) -> (x-y=w394:dbl)
            n313 = property on="History Plot" class="XYGraph (strict)"("X Scale.Range:Minimum"=w394) -> ()  [unwired: 2 in, 2 out]
          }
          event "15 min": Value Change {
            n314 = event-data() -> ()  [unwired: 1 in, 5 out]
            n315 = property on="History Plot" class="XYGraph (strict)"() -> ("X Scale.Range:Maximum"=w398:dbl)  [unwired: 2 in, 2 out]
            n316 = Subtract(x=w398, y=900) -> (x-y=w397:dbl)
            n317 = property on="History Plot" class="XYGraph (strict)"("X Scale.Range:Minimum"=w397) -> ()  [unwired: 2 in, 2 out]
          }
          event "30 min": Value Change {
            n318 = event-data() -> ()  [unwired: 1 in, 5 out]
            n319 = property on="History Plot" class="XYGraph (strict)"() -> ("X Scale.Range:Maximum"=w401:dbl)  [unwired: 2 in, 2 out]
            n320 = Subtract(x=w401, y=1800) -> (x-y=w400:dbl)
            n321 = property on="History Plot" class="XYGraph (strict)"("X Scale.Range:Minimum"=w400) -> ()  [unwired: 2 in, 2 out]
          }
          event "+1 hour": Value Change {
            n322 = event-data() -> ()  [unwired: 1 in, 5 out]
            n323 = property on="History Plot" class="XYGraph (strict)"() -> ("X Scale.Range:Minimum"=w404:dbl)  [unwired: 2 in, 2 out]
            n324 = Subtract(x=w404, y=3600) -> (x-y=w403:dbl)
            n325 = property on="History Plot" class="XYGraph (strict)"("X Scale.Range:Minimum"=w403) -> ()  [unwired: 2 in, 2 out]
          }
          event "Increase": Value Change {
            n326 = event-data() -> ()  [unwired: 1 in, 5 out]
            n327 = property on="History Plot" class="XYGraph (strict)"() -> ("Y Scale.Range:Maximum"=w408:dbl, "Y Scale.Range:Minimum"=w409:dbl)  [unwired: 2 in, 2 out]
            n328 = Subtract(x=w408, y=w409) -> (x-y=w406:dbl)
            n329 = Divide(x=w406, y=2) -> (x/y=w405:dbl)
            n330 = Add(x=w408, y=w405) -> (x+y=w410:dbl)
            n331 = Subtract(x=w409, y=w405) -> (x-y=w411:dbl)
            n332 = property on="History Plot" class="XYGraph (strict)"("Y Scale.Range:Maximum"=w410, "Y Scale.Range:Minimum"=w411) -> ()  [unwired: 2 in, 2 out]
          }
          event "Decrease": Value Change {
            n333 = event-data() -> ()  [unwired: 1 in, 5 out]
            n334 = property on="History Plot" class="XYGraph (strict)"() -> ("Y Scale.Range:Maximum"=w415:dbl, "Y Scale.Range:Minimum"=w416:dbl)  [unwired: 2 in, 2 out]
            n335 = Subtract(x=w415, y=w416) -> (x-y=w413:dbl)
            n336 = Divide(x=w413, y=4) -> (x/y=w412:dbl)
            n337 = Subtract(x=w415, y=w412) -> (x-y=w417:dbl)
            n338 = Add(x=w416, y=w412) -> (x+y=w418:dbl)
            n339 = property on="History Plot" class="XYGraph (strict)"("Y Scale.Range:Maximum"=w417, "Y Scale.Range:Minimum"=w418) -> ()  [unwired: 2 in, 2 out]
          }
          event "Up": Value Change {
            n340 = event-data() -> ()  [unwired: 1 in, 5 out]
            n341 = property on="History Plot" class="XYGraph (strict)"() -> ("Y Scale.Range:Maximum"=w422:dbl, "Y Scale.Range:Minimum"=w423:dbl)  [unwired: 2 in, 2 out]
            n342 = Subtract(x=w422, y=w423) -> (x-y=w420:dbl)
            n343 = Divide(x=w420, y=4) -> (x/y=w419:dbl)
            n344 = Add(x=w422, y=w419) -> (x+y=w424:dbl)
            n345 = Add(x=w423, y=w419) -> (x+y=w425:dbl)
            n346 = property on="History Plot" class="XYGraph (strict)"("Y Scale.Range:Maximum"=w424, "Y Scale.Range:Minimum"=w425) -> ()  [unwired: 2 in, 2 out]
          }
          event "Down": Value Change {
            n347 = event-data() -> ()  [unwired: 1 in, 5 out]
            n348 = property on="History Plot" class="XYGraph (strict)"() -> ("Y Scale.Range:Maximum"=w429:dbl, "Y Scale.Range:Minimum"=w430:dbl)  [unwired: 2 in, 2 out]
            n349 = Subtract(x=w429, y=w430) -> (x-y=w427:dbl)
            n350 = Divide(x=w427, y=4) -> (x/y=w426:dbl)
            n351 = Subtract(x=w429, y=w426) -> (x-y=w431:dbl)
            n352 = Subtract(x=w430, y=w426) -> (x-y=w432:dbl)
            n353 = property on="History Plot" class="XYGraph (strict)"("Y Scale.Range:Maximum"=w431, "Y Scale.Range:Minimum"=w432) -> ()  [unwired: 2 in, 2 out]
          }
          event "Submit Comment": Value Change {
            n354 = event-data() -> ()  [unwired: 1 in, 5 out]
            n355 = stacked-sequence {
              frame #0 {
                n356 = call "PDP Send User Comment.vi"("User Comment (press submit when done)") -> ()
              }
              frame #1 {
                n357 = local write "User Comment (press submit when done)"("") -> ()
              }
            }
          }
          event Timeout {
            n358 = event-data() -> ()  [unwired: 1 in, 2 out]
            n359 = local read "Clear Message Time"() -> (w442:i32)
            n360 = call "Get UNIX Time.vi"() -> ("UNIX_seconds_dbl"=w435:dbl)  [unwired: 10 in, 1 out]
            n361 = local read "Update At (sec)"() -> (w445:dbl)
            n362 = Greater Or Equal?(x=w435, y=w442) -> (x >= y?=w441:bool)
            n363 = Subtract(x=w445, y=w435) -> (x-y=w440:dbl)
            n364 = case shown="True" w441 {
              frame False {
              }
              frame True {
                n365 = local write "User Message"("") -> ()
              }
            }
            n366 = Greater Or Equal To 0?(x=w440) -> (x >= 0?=w444:bool)
            n367 = Equal?(x=w440, y=3) -> (x = y?=w438:bool)
            n368 = case shown="True" w444 {
              tunnel: w440 -> [_ w465]
              frame False {
                n369 = local read "NMR Tune Light"() -> (w463:bool)
                n370 = local read "Pause Light"() -> (w462:bool)
                n371 = Not Or(1:w463, 2:w462) -> (0:w464:bool)
                n372 = property on="Next Update" class="DigNum (strict)"("Visible"=w464) -> ()  [unwired: 2 in, 2 out]
              }
              frame True {
                "Next Update" <- w465
              }
            }
            n373 = And(x=w438, y="auto_switch_NMR_chan") -> (x .and. y?=w436:bool)
            n374 = case shown="True" w436 {
              frame False {
              }
              frame True {
                n375 = property on="NMR Channel" class="LstBox (strict)"() -> ("Item Names"=w447:string[])  [unwired: 2 in, 2 out]
                n376 = local read "NMR Channel"() -> (w448:i32)
                n377 = Array Size(array=w447) -> (size(s)=w446:i32)
                n378 = while {
                  tunnel: w446 -> [w459]
                  shift-right: [w450] -> w449
                  shift-left: w448 -> [w460]
                  tunnel: w448 -> [w455]
                  stop <- w451 stop-if-true
                  n379 = Increment(x=w460) -> (x+1=w457:i32)
                  n380 = Not Equal?(x=w457, y=w459) -> (x != y?=w458:bool)
                  n381 = Select(t=w457, s=w458, f=0) -> (s? t:f=w450:i32)
                  n382 = Equal?(x=w455, y=w450) -> (x = y?=w453:bool)
                  n383 = Index Array(array="sel_auto_sw", index=w450) -> (element=w452:bool)
                  n384 = Or(x=w453, y=w452) -> (x .or. y?=w451:bool)
                }
                n385 = property on="NMR Channel" class="LstBox (strict)"("Val(Sgnl)"=w449) -> ()  [unwired: 2 in, 2 out]
              }
            }
            n386 = property on="Error" class="Bool (strict)"() -> ("Blinking"=w443:bool)  [unwired: 2 in, 2 out]
            n387 = case shown="True" w443 {
              frame False {
              }
              frame True {
                n388 = call <vilib>:"Beep.vi"() -> ()  [unwired: 12 in]
              }
            }
          }
        }
      }
    }
    frame #2 {
    }
  }
